vi "Convert Profile Point to String.vi"(7 "Point String":string, 11 "Point Cluster":T1) -> (3 "Point Cluster Out":T1, 5 "Point String Out":string)   [LabVIEW 2016]
uses:
  RoboRio code/TypeDef/CLUSTER_Drive_Point Specification.ctl
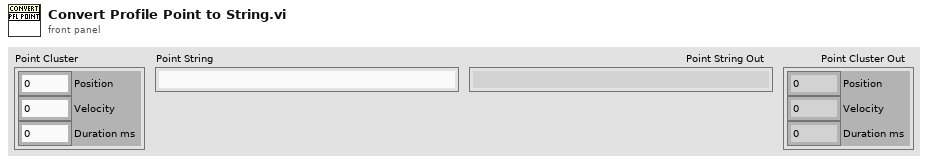
[diagram p1: front panel]
types:
  T1 = typedef "CLUSTER_Drive_Point Specification.ctl" = cluster{"Position":dbl, "Velocity":dbl, "Duration ms":u8}
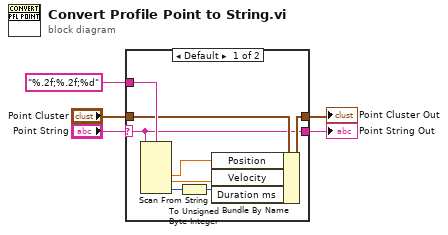
[diagram p0: block diagram]
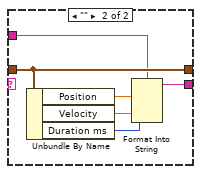
[diagram p2: hidden frame]
diagram:
  n1 = case shown="Default" "Point String" {
    selector: "Point String" -> [w6 _]
    tunnel: "Point Cluster" -> [w12 w15]
    tunnel: [w6 w16] -> w4
    tunnel: [w11 w15] -> w2
    tunnel: "%.2f;%.2f;%d" ("format string") -> [w13 w14]
    frame Default {
      n2 = Scan From String(format string=w13, input string=w6) -> (output 1=w10:dbl, output 2=w9:dbl, output 3=w8:i32)  [unwired: 5 in, 3 out]
      n3 = To Unsigned Byte Integer(number=w8) -> (unsigned 8bit integer=w7:u8)
      n4 = Bundle By Name(cluster=w12, "Position"=w10, "Velocity"=w9, "Duration ms"=w7) -> (w11:T1)
    }
    frame "" {
      n5 = Unbundle By Name(w15) -> ("Position"=w19:dbl, "Velocity"=w18:dbl, "Duration ms"=w17:u8)
      n6 = Format Into String(format string=w14, w19, w18, w17) -> (resulting string=w16:string)  [unwired: 2 in, 1 out]
    }
  }
  "Point Cluster Out" <- w2
  "Point String Out" <- w4
